vi "Repeat Message Async.vi"(4 "First Immediate (F)":bool, 6 "Period ms":u32, 7 "High Priority (F)":bool, 8 "Repeat Message Control":refnum<class "Repeat Message Control.lvclass">, 9 "Data":variant, 10 "ID":string, 11 "MessageQ in":refnum<class "MessageQ.lvclass">) -> ()   [LabVIEW 2020, in "Volatus.lvlib" / "MessageQ.lvclass"]
uses:
  MessageQ.lvclass
  Repeat Message Control/Repeat Message Control.lvclass
  MessageQ.lvclass/MessageQ.ctl
  Repeat Message Control/Repeat Message Control.lvclass/Repeat Message Control.ctl
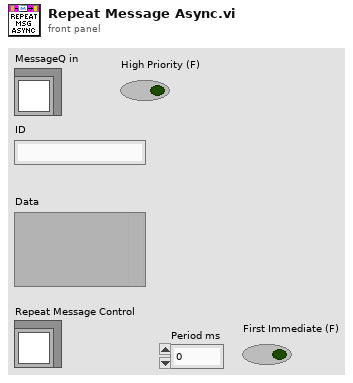
[diagram p1: front panel]
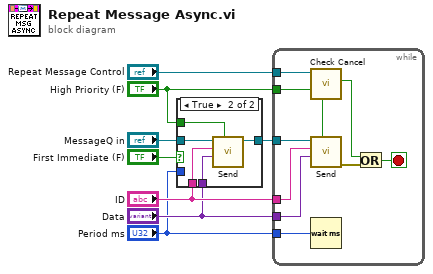
[diagram p0: block diagram]
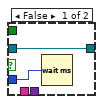
[diagram p2: hidden frame]
diagram:
  n1 = case shown="True" "First Immediate (F)" {
    tunnel: "MessageQ in" -> [w10 w15]
    tunnel: [w10 w14] -> w6
    tunnel: "High Priority (F)" -> [_ w13]
    tunnel: "ID" -> [_ w12]
    tunnel: "Data" -> [_ w11]
    tunnel: "Period ms" -> [w9 _]
    frame False {
      n2 = Wait (ms)(milliseconds to wait=w9) -> ()  [unwired: 1 out]
    }
    frame True {
      n3 = call "Send.vi"("High Priority (F)"=w13, "Data"=w11, "ID"=w12, "MessageQ in"=w15) -> ("MessageQ out"=w14:refnum<class "MessageQ.lvclass">)  [unwired: 6 in, 1 out]
    }
  }
  n4 = while {
    tunnel: w6 -> [w22]
    tunnel: "ID" -> [w20]
    tunnel: "Data" -> [w19]
    tunnel: "Period ms" -> [w24]
    tunnel: "High Priority (F)" -> [w21]
    tunnel: "Repeat Message Control" -> [w23]
    stop <- w16 stop-if-true
    n5 = call "Check Cancel.vi"("Repeat Message Control in"=w23) -> ("Cancel"=w17:bool)  [unwired: 10 in]
    n6 = call "Send.vi"("High Priority (F)"=w21, "Data"=w19, "ID"=w20, "MessageQ in"=w22) -> ("error out"=w18:errorcluster)  [unwired: 6 in, 1 out]
    n7 = Wait (ms)(milliseconds to wait=w24) -> ()  [unwired: 1 out]
    n8 = Or(x=w17, y=w18) -> (x .or. y?=w16:bool)
  }
